vi "GitStatus.vi"(6 "UsePopup(T)":bool=TRUE, 8 "error in (no error)":errorcluster, 11 "Directory (leave empty for relative)":path) -> (0 "error out":errorcluster, 3 "directory out":path, 5 "Git Ok?(t)":bool, 7 "Cancel?(t)":bool caption="STOP")   [LabVIEW 2018]
panel:
  out "standard output":string
  out "git status":string[](array[string])
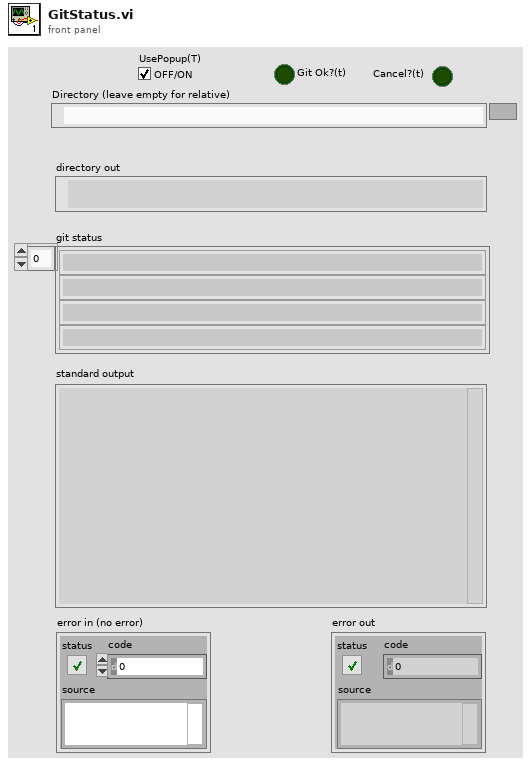
[diagram p1: front panel]
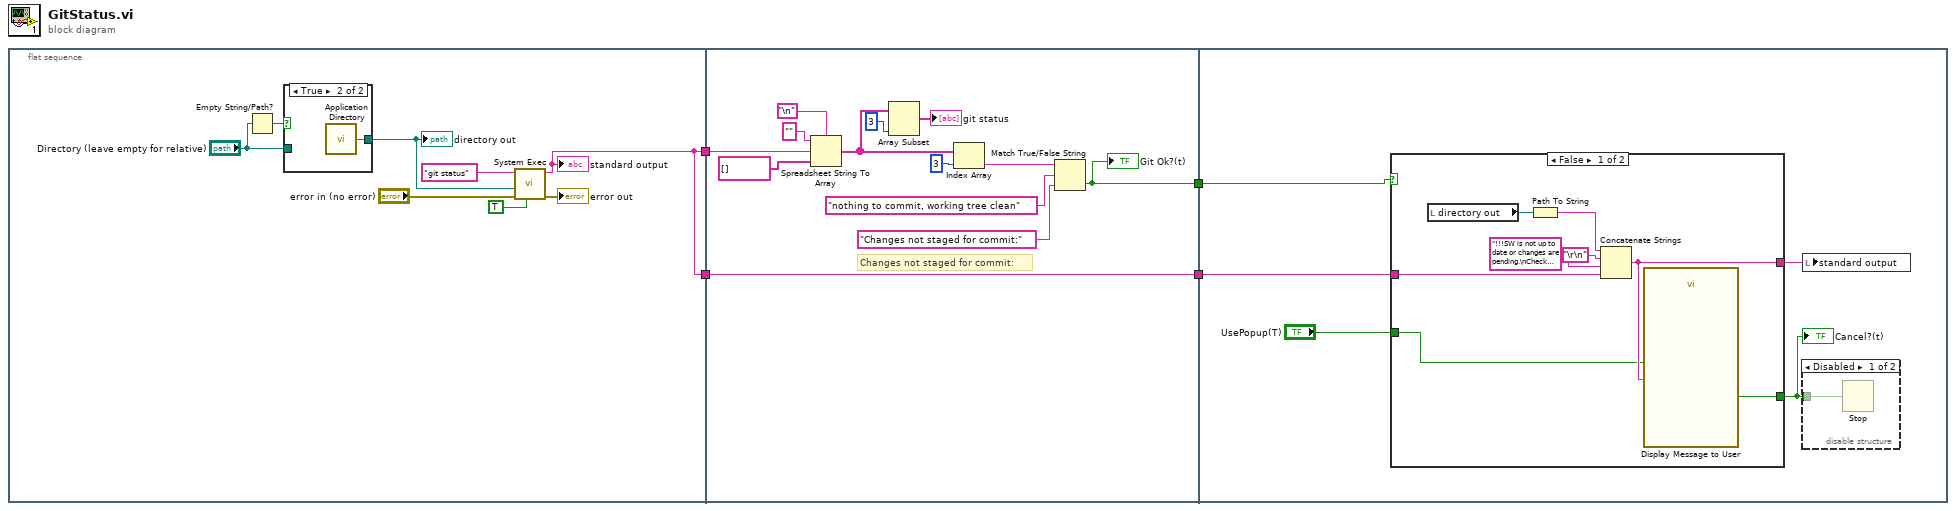
[diagram p0: block diagram]
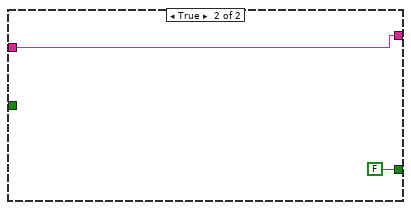
[diagram p4: hidden frame]
diagram:
  n1 = flat-sequence {
    tunnel: [w5] -> w4
    tunnel: [w5] -> w2
    tunnel: w4 -> [w17]
    tunnel: [w16] -> w3
    tunnel: w2 -> [w15]
    tunnel: [w15] -> w1
    tunnel: w3 -> [w29]
    tunnel: w1 -> [w32]
    frame #0 {
      n2 = Empty String/Path?(string/path="Directory (leave empty for relative)") -> (empty?=w6:bool)
      n3 = case shown="True" w6 {
        tunnel: [w13 w14] -> w8
        tunnel: "Directory (leave empty for relative)" -> [w13 _]
        frame False {
        }
        frame True {
          n4 = call <vilib>:"Application Directory.vi"() -> ("Application Directory"=w14:path)
        }
      }
      "directory out" <- w8
      n5 = call <vilib>:"System Exec.vi"("run minimized? (F)"=TRUE, "error in (no error)"="error in (no error)", "working directory"=w8, "command line"="git status") -> ("error out"=→"error out":errorcluster, "standard output"=w5:string)  [unwired: 4 in, 2 out]
      "standard output" <- w5
    }
    frame #1 {
      # "Changes not staged for commit:"
      n6 = Spreadsheet String To Array(delimiter (Tab)="\n", format string="", spreadsheet string=w17, array type (2D Dbl)=string[] []) -> (array=w26:string[])
      n7 = Array Subset(array=w26, length=3) -> (→"git status":string[])  [unwired: 1 in]
      n8 = Index Array(array=w26, index=3) -> (element=w27:string)
      n9 = Match True/False String(2:"Changes not staged for commit:" ("false string"), 3:"nothing to commit, working tree clean" ("false string"), 4:w27) -> (0:w16:bool)  [unwired: 1 out]
      "Git Ok?(t)" <- w16
    }
    frame #2 {
      n10 = case shown="False" w29 {
        tunnel: [w39 w43] -> w31
        tunnel: w32 -> [w40 w43]
        tunnel: [w38 FALSE ("STOP")] -> w30
        tunnel: "UsePopup(T)" -> [w34 _]
        frame False {
          n11 = local read "directory out"() -> (w37:path)
          n12 = Path To String(path=w37) -> (string=w36:string)
          n13 = Concatenate Strings(w36, "\r\n", "!!!SW is not up to date or changes are pending.\nCheck the message and correct the issue using Github!!", w40) -> (w39:string)
          n14 = call "Display Message to User"("Enable"=w34, "Message"=w39) -> ("STOP"=w38:bool)  [unwired: 8 in, 1 out]
        }
        frame True {
        }
      }
      "Cancel?(t)" <- w30
      n15 = local write "standard output"(w31) -> ()
      n16 = disable-structure shown="Disabled" {
        disable-tunnel: w30 -> [w33 _]
        frame Disabled {
          n17 = Stop(stop? (T)=w33) -> ()
        }
        frame Enabled {
        }
      }
    }
  }
